vi "file_check_label.vi"(0 "base path":path, 1 "prefix":string, 2 "index":dbl, 3 "Loop Data Labels":string[](array[string])=["Vap Mass Flow", "Liq Mass Flow", "DP", "Liq Tank P", "LiqTank T", "Sep P", "SepT", "Liq In P", "Liq In T", "Vap Tank P", "Vap Tank T", "Dev Section P", "Dev Section T", "Up TS P", "Up TS T", "Low TS P", "Low TS T", "Cond Top T", "Evap Top T", "Cond Bot T", "Evap Bot T", "Win 3-4 P", "Top Heat T", "Bot Heat T"], 4 "task name":string) -> (5 "dup path":path, 6 "error out":errorcluster)   [LabVIEW 2015]
uses:
  <vilib>/Utility/file.llb/Write Delimited Spreadsheet (string).vi
  <vilib>/Utility/sysdir.llb/System Directory Type.ctl
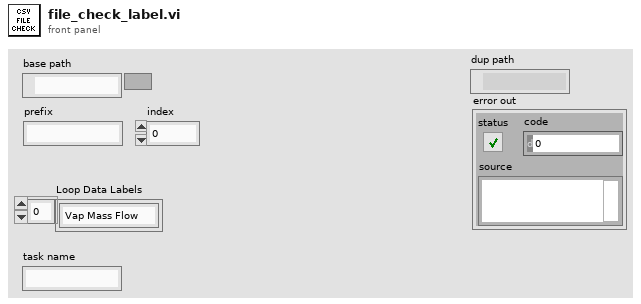
[diagram p1: front panel]
types:
  T1 = typedef "System Directory Type.ctl" = i32
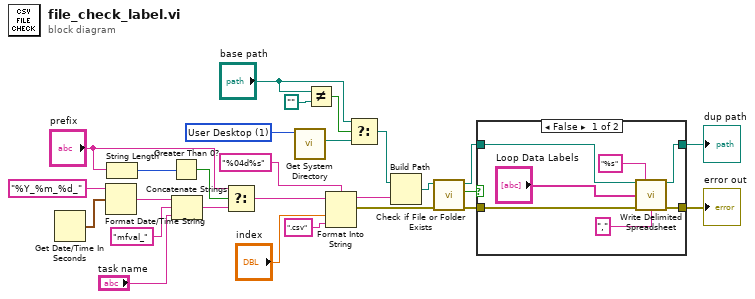
[diagram p0: block diagram]
diagram:
  w16 = T1 1 items=["User Home"=0, "User Desktop"=1, "User Documents"=2, "User Application Data"=3, "User Preferences"=4, "User Temporary"=5, "Public Documents"=6, "Public Application Data"=7, "Public Preferences"=8, "Public Cache"=13, "System Core Libraries"=9, "System Installed Libraries"=10, "Application Files"=11, "Boot Volume Root"=12] ("system directory type")
  n1 = Get Date/Time In Seconds() -> (seconds since 1Jan1904=w11:timestamp)
  n2 = Format Date/Time String(time format string (%c)="%Y_%m_%d_", seconds (now)=w11) -> (date/time string=w9:string)  [unwired: 1 in]
  n3 = String Length(string="prefix") -> (length=w15:i32)
  n4 = Greater Than 0?(x=w15) -> (x > 0?=w14:bool)
  n5 = Concatenate Strings(w9, "mfval_" ("string"), "task name") -> (w8:string)
  n6 = Select(t="prefix", s=w14, f=w8) -> (s? t:f=w12:string)
  n7 = call <vilib>:"Get System Directory.vi"("system directory type"=w16) -> ("system directory"=w4:path)  [unwired: 10 in]
  n8 = Not Equal?(x="base path", y=path "") -> (x != y?=w5:bool)
  n9 = Format Into String(format string="%04d%s", initial string=w12, "index", ".csv") -> (resulting string=w27:string, error out=w25:errorcluster)  [unwired: 1 in]
  n10 = Select(t="base path", s=w5, f=w4) -> (s? t:f=w6:path)
  n11 = Build Path(base path=w6, name or relative path=w27) -> (appended path=w26:path)
  n12 = call <vilib>:"Check if File or Folder Exists.vi"("error in (no error)"=w25, "path"=w26) -> ("error out"=w22:errorcluster, "file or folder exists?"=w24:bool, "dup path"=w23:path)  [unwired: 7 in]
  n13 = case shown="False" w24 {
    tunnel: [w34 w36] -> w18
    tunnel: w23 -> [w31 w36]
    tunnel: [w33 w35] -> w17
    tunnel: w22 -> [w32 w35]
    frame False {
      n14 = call-poly <vilib>:"Write Delimited Spreadsheet.vi"("file path (dialog if empty)"=w31, "format (%s)"="%s", "1D data"="Loop Data Labels", "error in (no error)"=w32, "delimiter (\\t)"="," ("delimiter (\\t)")) -> ("new file path (Not A Path if cancelled)"=w34:path, "error out"=w33:errorcluster)  [unwired: 9 in]
    }
    frame True {
    }
  }
  "dup path" <- w18
  "error out" <- w17
